vi "4310 DMM Configure and Start.vi"(0 "IVI Refnum in":refnum<k15>="DMM" caption="Device Name", 1 "Slope":T4=enum."Falling Edge", 2 "Number of Samples in":i32=1000, 3 "Sample Rate":dbl=20000.0, 4 "Sample Clock Source":tag="OnboardClock", 5 "error in (no error)":errorcluster, 6 "Range":dbl=1000.0 format="%.2p", 7 "Terminal Configuration":i32(ring)=-1 items=["default"=-1, "RSE"=10083, "NRSE"=10078, "Differential"=10106, "Pseudodifferential"=12529], 8 "Function":T1, 9 "Min Voltage":dbl=-10.0, 10 "Resolution in Digits":T2=3.5 items=["3 1/2"=3.5, "4 1/2"=4.5, "5 1/2"=5.5, "6 1/2"=6.5, "7 1/2"=7.5], 11 "Max Voltage":dbl=10.0, 12 "Trigger Source":T3=enum."TTL 0", 13 "Physical Channel":tag="4310/ai0:7") -> (14 "IVI Refnum out":refnum<k15>, 15 "task out":refnum<k21>, 17 "Number of Samples out":i32, 19 "error out":errorcluster)   [LabVIEW 2019]
uses:
  <instrlib>/niDMM/nidmm.llb/niDMM Slope.ctl
  <instrlib>/niDMM/nidmm.llb/niDMM Trigger.ctl
  <instrlib>/niDMM/nidmm.llb/niDMM Resolution in Digits.ctl
  <instrlib>/niDMM/nidmm.llb/niDMM Function.ctl
  <instrlib>/niDMM/nidmm.llb/niDMM Sample Trigger.ctl
  <instrlib>/niDMM/nidmm.llb/niDMM Configure Measurement Digits.vi
  <vilib>/DAQmx/create/channels.llb/DAQmx Create Channel (AI-Voltage-Basic).vi
  <vilib>/DAQmx/configure/timing.llb/DAQmx Timing (Sample Clock).vi
  <vilib>/DAQmx/configure/events/hardwareSignals.llb/DAQmx Export Signal (Most Signals).vi
  <vilib>/NI_Real-Time Target Support.lvlib
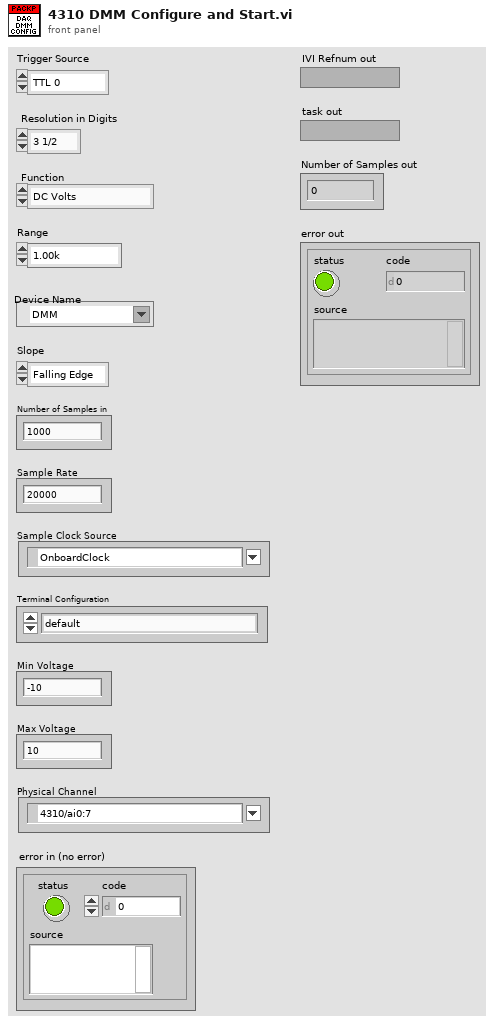
[diagram p1: front panel]
types:
  T1 = typedef "niDMM Function.ctl" = enum16{"DC Volts", "AC Volts", "DC Current", "AC Current", "2-wire Resistance", "4-wire Resistance", "Diode", "Frequency", "Period", "AC Volts DC Coupled", "Capacitance", "Inductance", "Temperature"}
  T2 = typedef "niDMM Resolution in Digits.ctl" = dbl
  T3 = typedef "niDMM Trigger.ctl" = enum16{"Immediate", "External", "TTL 0", "TTL 1", "TTL 2", "TTL 3", "TTL 4", "TTL 5", "TTL 6", "Software", "TTL 7", "PXI Star", "LBR Trig 1", "Aux Trig 1"}
  T4 = typedef "niDMM Slope.ctl" = enum16{"Rising Edge", "Falling Edge"}
  T5 = typedef "niDMM Sample Trigger.ctl" = enum16{"Immediate", "External", "TTL 0", "TTL 1", "TTL 2", "TTL 3", "TTL 4", "TTL 5", "TTL 6", "Interval", "Software", "TTL 7", "PXI Star", "LBR Trig 1", "Aux Trig 1"}
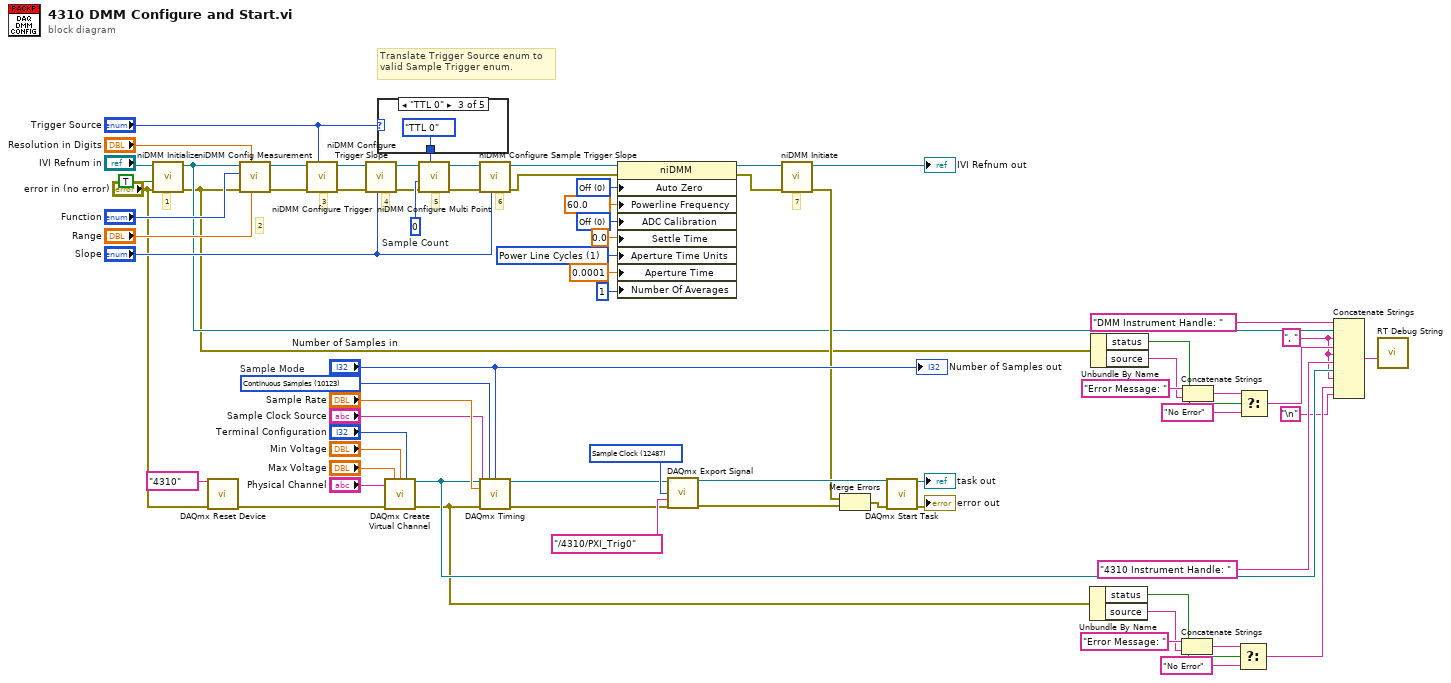
[diagram p0: block diagram]
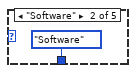
[diagram p3: hidden frame]
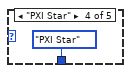
[diagram p4: hidden frame]
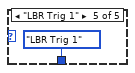
[diagram p5: hidden frame]
diagram:
  w15 = ", "
  w71 = 0 items=["Auto"=-1, "Off"=0, "On"=1, "Once"=2] ("Configuration:Measurement Options:Auto Zero")
  w70 = 60.0 items=["50 Hz"=50.0, "60 Hz"=60.0] ("Configuration:Measurement Options:Powerline Frequency")
  w69 = 0 items=["Auto"=-1, "Off"=0, "On"=1] ("Configuration:Measurement Options:ADC Calibration")
  w67 = 1 items=["Seconds", "Power Line Cycles"] ("Configuration:Advanced:Aperture Time Units")
  w60 = 12487 items=["AI Convert Clock"=12484, "10MHz Reference Clock"=12536, "20MHz Timebase Clock"=12486, "Sample Clock"=12487, "Advance Trigger"=12488, "Reference Trigger"=12490, "Start Trigger"=12491, "Advance Complete Event"=12492, "AI Hold Complete Event"=12493, "Counter Output Event"=12494, "Change Detection Event"=12511, "Watchdog Timer Expired Event"=12512] ("signal")
  w48 = 10123 items=["Finite Samples"=10178, "Continuous Samples"=10123, "Hardware Timed Single Point"=12522]  # Sample Mode
  w41 = 0  # Sample Count
  # "4"
  # "6"
  # "5"
  # "7"
  # "Translate Trigger Source enum to\nvalid Sample Trigger enum."
  # "3"
  # "2"
  # "1"
  n1 = call <instrlib>:"niDMM Initialize.vi"("error in (no error)"="error in (no error)", "Reset"=TRUE, "Instrument Descriptor"="IVI Refnum in") -> ("error out"=w25:errorcluster, "instrument handle out"=w26:refnum<k15>)  [unwired: 7 in]
  n2 = call <vilib>:"DAQmx Reset Device.vi"("device in"=tag "4310", "error in"="error in (no error)") -> ("error out"=w2:errorcluster)  [unwired: 13 in]
  n3 = call-poly <instrlib>:"niDMM Config Measurement.vi"("Range"="Range", "Resolution in Digits"="Resolution in Digits", "error in (no error)"=w25, "Function"="Function", "instrument handle"=w26) -> ("error out"=w33:errorcluster, "instrument handle out"=w32:refnum<k15>)  [unwired: 5 in]
  n4 = call <instrlib>:"niDMM Configure Trigger.vi"("Trigger Source"="Trigger Source", "error in (no error)"=w33, "instrument handle"=w32) -> ("error out"=w35:errorcluster, "instrument handle out"=w34:refnum<k15>)  [unwired: 7 in]
  n5 = call <instrlib>:"niDMM Configure Trigger Slope.vi"("Slope"="Slope", "error in (no error)"=w35, "instrument handle"=w34) -> ("error out"=w37:errorcluster, "instrument handle out"=w36:refnum<k15>)  [unwired: 7 in]
  n6 = case shown="\"TTL 0\"" "Trigger Source" {
    selector: "Trigger Source" -> [w72 _ _ _ _]
    tunnel: [w72 niDMM_Sample_Trigger."Software" ("Sample Trigger") niDMM_Sample_Trigger."TTL 0" ("Sample Trigger") niDMM_Sample_Trigger."PXI Star" ("Sample Trigger") niDMM_Sample_Trigger."LBR Trig 1" ("Sample Trigger")] -> w44
    frame "Immediate", Default {
    }
    frame "Software" {
    }
    frame "TTL 0" {
    }
    frame "PXI Star" {
    }
    frame "LBR Trig 1" {
    }
  }
  n7 = call-poly <vilib>:"DAQmx Create Virtual Channel.vi"("maximum value"="Max Voltage", "minimum value"="Min Voltage", "input terminal configuration"="Terminal Configuration", "physical channels"="Physical Channel", "error in"=w2) -> ("task out"=w16:refnum<k21>, "error out"=w9:errorcluster)  [unwired: 9 in]
  n8 = call <instrlib>:"niDMM Configure Multi Point.vi"("Sample Trigger"=w44, "error in (no error)"=w37, "Sample Count"=w41, "instrument handle"=w36) -> ("error out"=w39:errorcluster, "instrument handle out"=w38:refnum<k15>)  [unwired: 6 in]
  n9 = call <instrlib>:"niDMM Configure Sample Trigger Slope.vi"("Slope"="Slope", "error in (no error)"=w39, "instrument handle"=w38) -> ("error out"=w63:errorcluster, "instrument handle out"=w45:refnum<k15>)  [unwired: 7 in]
  n10 = call-poly <vilib>:"DAQmx Timing.vi"("task/channels in"=w16, "sample mode"=w48, "samples per channel"="Number of Samples in", "rate"="Sample Rate", "source"="Sample Clock Source", "error in"=w9) -> ("task out"=w57:refnum<k21>, "error out"=w59:errorcluster)  [unwired: 8 in]
  n11 = property class="niDMM"(reference=w45, error in=w63, "Auto Zero"=w71, "Powerline Frequency"=w70, "ADC Calibration"=w69, "Settle Time"=0.0 ("Configuration:Advanced:Settle Time"), "Aperture Time Units"=w67, "Aperture Time"=0.0001 ("Configuration:Advanced:Aperture Time"), "Number Of Averages"=1 ("Configuration:Advanced:Number Of Averages")) -> (reference out=w62:refnum<k15>, error out=w64:errorcluster)
  n12 = call-poly <vilib>:"DAQmx Export Signal.vi"("task/channels in"=w57, "signal"=w60, "output terminal"=tag "/4310/PXI_Trig0", "error in"=w59) -> ("task out"=w58:refnum<k21>, "error out"=w6:errorcluster)  [unwired: 10 in]
  n13 = call <instrlib>:"niDMM Initiate.vi"("error in (no error)"=w64, "instrument handle"=w62) -> ("error out"=w28:errorcluster, "instrument handle out"=→"IVI Refnum out":refnum<k15>)  [unwired: 8 in]
  n14 = Merge Errors(w28, w6) -> (w5:errorcluster)
  n15 = call <vilib>:"DAQmx Start Task.vi"("task/channels in"=w58, "error in"=w5) -> ("task out"=→"task out":refnum<k21>, "error out"=→"error out":errorcluster)  [unwired: 12 in]
  n16 = Unbundle By Name(w9) -> ("status"=w14:bool, "source"=w12:string)
  n17 = Unbundle By Name(w25) -> ("status"=w23:bool, "source"=w21:string)
  n18 = Concatenate Strings("Error Message: " ("String to write"), w12) -> (w11:string)
  n19 = Concatenate Strings("Error Message: " ("String to write"), w21) -> (w20:string)
  n20 = Select(t=w11, s=w14, f="No Error") -> (s? t:f=w8:string)
  n21 = Select(t=w20, s=w23, f="No Error") -> (s? t:f=w18:string)
  n22 = Concatenate Strings("DMM Instrument Handle: " ("String to write"), w26, w15, w18, w15, "4310 Instrument Handle: " ("String to write"), w16, w15, w8, "\n") -> (w24:string)
  n23 = call <vilib>:"RT Debug String.vi"("String to write"=w24) -> ()  [unwired: 10 in, 1 out]
  "Number of Samples out" <- "Number of Samples in"
